vi "Display.vi"(11 "Array in":i32[](array[numeric])) -> (3 "Array out":i32[](array[numeric]))   [LabVIEW 2020]
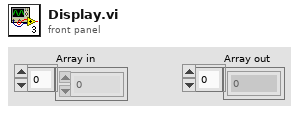
[diagram p1: front panel]
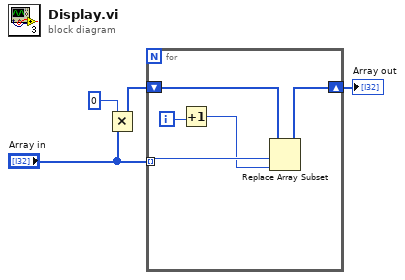
[diagram p0: block diagram]
diagram:
  n1 = Multiply(x=0, y="Array in") -> (x*y=w2:i32[])
  n2 = for {
    tunnel: "Array in" -> [w7] mode=indexing
    shift-right: [w5] -> w4
    shift-left: w2 -> [w8]
    i -> [w9]
    n3 = Increment(x=w9) -> (x+1=w6:i32)
    n4 = Replace Array Subset(array=w8, new element=w6, index=w7) -> (w5:i32[])
  }
  "Array out" <- w4
